vi "Set Event Measurement Properties.vi"(8 "error in (no error)":errorcluster, 10 "measurement":T1={"Name"="", "Bitfile name"="", "Window"="", "Polarity"=enum."Active high"}, 11 "Item Ref in":T3 format="%.0x") -> (0 "error out":errorcluster, 2 "failed":bool, 3 "Item Ref out":T3 format="%.0x")   [LabVIEW 2015, in "Engine Simulation Toolkit System Explorer.lvlib"]
uses:
  Engine Simulation Toolkit System Explorer.lvlib
  <vilib>/NI Veristand/Custom Device API/Custom Device Item Ref.ctl
  Event Timing Measurement.ctl
  Polarity.ctl
  Shared/Properties.vi
  <vilib>/NI Veristand/Custom Device Tools/Custom Device Utility Library/NI VeriStand - Search for Item by Property.vi
  <vilib>/NI Veristand/Custom Device API/Set Item Property (String).vi
  <vilib>/NI Veristand/Custom Device API/Set Item Property (U16).vi
  <vilib>/NI Veristand/Custom Device API/Custom Device API.lvlib
  Shared/Engine Simulation Toolkit Shared.lvlib
  <vilib>/NI Veristand/Custom Device Tools/Custom Device Utility Library/Custom Device Utility Library.lvlib
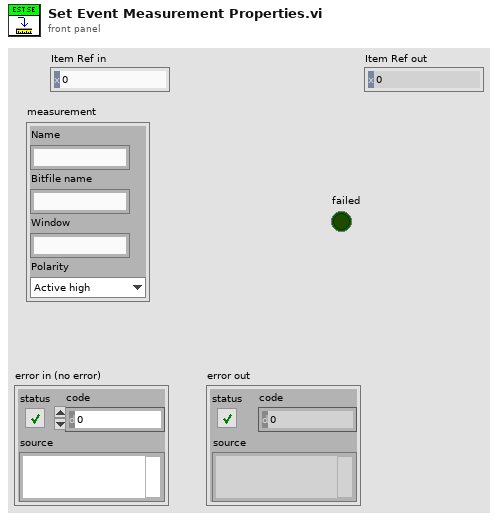
[diagram p1: front panel]
types:
  T1 = typedef "Engine Simulation Toolkit System Explorer.lvlib/Event Timing Measurement.ctl" = cluster{"Name":string, "Bitfile name":string, "Window":string, "Polarity":T2}
  T2 = typedef "Engine Simulation Toolkit System Explorer.lvlib/Polarity.ctl" = enum16{"Active low", "Active high"}
  T3 = typedef "Custom Device API.lvlib/Custom Device Item Ref.ctl" = u64
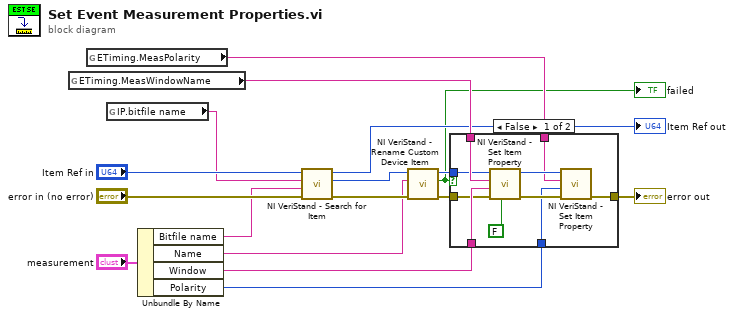
[diagram p0: block diagram]
diagram:
  n1 = global read "Properties.vi" "ETiming.MeasWindowName"() -> (w15:string)
  n2 = global read "Properties.vi" "ETiming.MeasPolarity"() -> (w8:string)
  n3 = global read "Properties.vi" "IP.bitfile name"() -> (w6:string)
  n4 = Unbundle By Name("measurement") -> ("Bitfile name"=w7:string, "Name"=w2:string, "Window"=w10:string, "Polarity"=w9:T2)
  n5 = call-poly <vilib>:"NI VeriStand - Search for Item.vi"("error in"="error in (no error)", "Property Value"=w7, "Property Name"=w6, "Section Ref in"="Item Ref in") -> ("error out"=w13:errorcluster, "Item Ref"=w4:T3, "Section Ref out"=→"Item Ref out":T3)  [unwired: 4 in, 1 out]
  n6 = call <vilib>:"NI VeriStand - Rename Custom Device Item.vi"("error in (no error)"=w13, "New Name"=w2, "Item Ref in"=w4) -> ("error out"=w5:errorcluster, "Request invalid?"=w1:bool, "Item Ref out"=w3:T3)  [unwired: 6 in]
  "failed" <- w1
  n7 = case shown="False" w1 {
    tunnel: [w26 w28] -> w16
    tunnel: w15 -> [w24 _]
    tunnel: w10 -> [w23 _]
    tunnel: w9 -> [w22 _]
    tunnel: w8 -> [w21 _]
    tunnel: w5 -> [w20 w28]
    tunnel: w3 -> [w19 _]
    frame False {
      n8 = call-poly <vilib>:"NI VeriStand - Set Item Property.vi"("Binary String (T)"=FALSE, "error in (no error)"=w20, "Value"=w23, "Property Name"=w24, "Item Ref in"=w19) -> ("error out"=w27:errorcluster, "Item Ref out"=w25:T3)  [unwired: 4 in, 1 out]
      n9 = call-poly <vilib>:"NI VeriStand - Set Item Property.vi"("error in (no error)"=w27, "Value"=w22, "Property Name"=w21, "Item Ref in"=w25) -> ("error out"=w26:errorcluster)  [unwired: 5 in, 2 out]
    }
    frame True {
    }
  }
  "error out" <- w16
